vi "CallRosco_v2.vi"(6 "StopLV":bool, 8 "error in (no error)":errorcluster, 9 "ROSCO Params in":T3, 11 "ArrayPairs":T1={"iStatus"={"Index"=0, "Value"=0.0}, "TIME"={"Index"=1, "Value"=0.0}, "DT"={"Index"=2, "Value"=0.0}, "BL_PITCH"={"Index"=3, "Value"=0.0}, "VS_MECHGENPWR"={"Index"=13, "Value"=0.0}, "VS_GENPWR"={"Index"=14, "Value"=0.0}, "GEN_SPEED"={"Index"=19, "Value"=0.0}, "ROTOR_SPEED"={"Index"=20, "Value"=0.0}, "GENTQMEAS"={"Index"=22, "Value"=0.0}, "Y_M"={"Index"=23, "Value"=0.0}, "HORWINDV"={"Index"=26, "Value"=0.0}, "ROOTMOOP1"={"Index"=29, "Value"=0.0}, "ROOTMOOP2"={"Index"=30, "Value"=0.0}, "BL_PITCH2"={"Index"=32, "Value"=0.0}, "BL_PITCH3"={"Index"=33, "Value"=0.0}, "ROOTMOOP3"={"Index"=31, "Value"=0.0}, "AVCMSG_SIZE"={"Index"=48, "Value"=0.0}, "INFILE_SIZE "={"Index"=49, "Value"=0.0}, "OUTFILE_SIZE "={"Index"=50, "Value"=0.0}, "FA_ACC"={"Index"=52, "Value"=0.0}, "NUM_BLADES"={"Index"=60, "Value"=0.0}, "OUT_BL_PITCH"={"Index"=44, "Value"=0.0}, "OUT_TORQUE"={"Index"=46, "Value"=0.0}, "OUT_AERODYN_TQ"={"Index"=89, "Value"=0.0}}) -> (0 "error out":errorcluster, 1 "ROSCO Params out":T3, 4 "ArrayPairs 2":T1={"iStatus"={"Index"=0, "Value"=0.0}, "TIME"={"Index"=1, "Value"=0.0}, "DT"={"Index"=2, "Value"=0.0}, "BL_PITCH"={"Index"=3, "Value"=0.0}, "VS_MECHGENPWR"={"Index"=13, "Value"=0.0}, "VS_GENPWR"={"Index"=14, "Value"=0.0}, "GEN_SPEED"={"Index"=19, "Value"=0.0}, "ROTOR_SPEED"={"Index"=20, "Value"=0.0}, "GENTQMEAS"={"Index"=22, "Value"=0.0}, "Y_M"={"Index"=23, "Value"=0.0}, "HORWINDV"={"Index"=26, "Value"=0.0}, "ROOTMOOP1"={"Index"=29, "Value"=0.0}, "ROOTMOOP2"={"Index"=30, "Value"=0.0}, "BL_PITCH2"={"Index"=32, "Value"=0.0}, "BL_PITCH3"={"Index"=33, "Value"=0.0}, "ROOTMOOP3"={"Index"=31, "Value"=0.0}, "AVCMSG_SIZE"={"Index"=48, "Value"=0.0}, "INFILE_SIZE "={"Index"=49, "Value"=0.0}, "OUTFILE_SIZE "={"Index"=50, "Value"=0.0}, "FA_ACC"={"Index"=52, "Value"=0.0}, "NUM_BLADES"={"Index"=60, "Value"=0.0}, "OUT_BL_PITCH"={"Index"=44, "Value"=0.0}, "OUT_TORQUE"={"Index"=46, "Value"=0.0}, "OUT_AERODYN_TQ"={"Index"=89, "Value"=0.0}})   [LabVIEW 2018]
uses:
  Clusters/RoscoParams.ctl
  Clusters/ArrayPairs.ctl
  Clusters/SwapArrayCluster.ctl
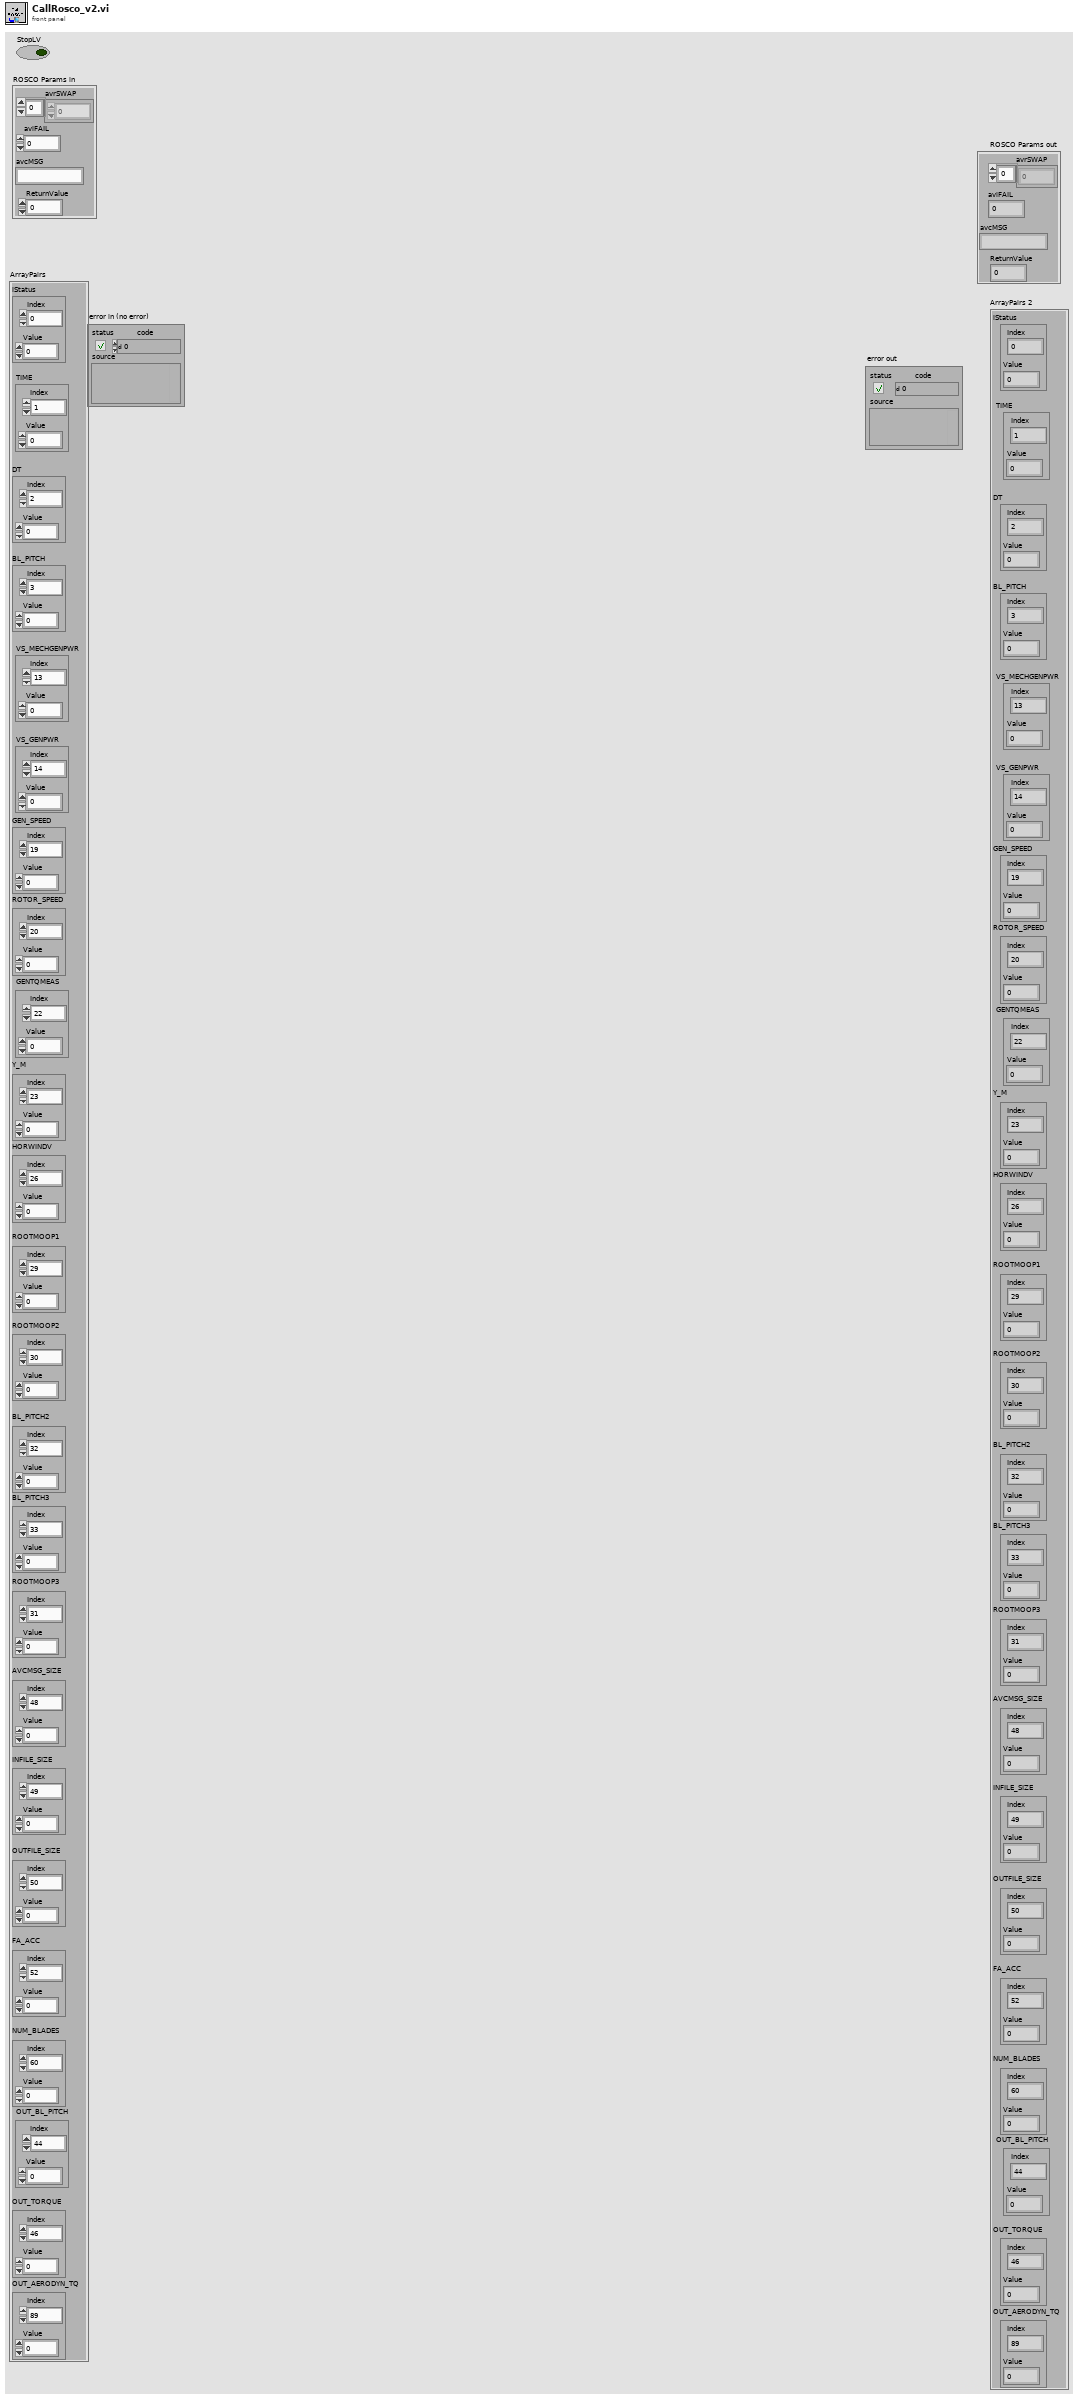
[diagram p1: front panel]
types:
  T1 = typedef "ArrayPairs.ctl" = cluster{"iStatus":T2, "TIME":T2, "DT":T2, "BL_PITCH":T2, "VS_MECHGENPWR":T2, "VS_GENPWR":T2, "GEN_SPEED":T2, "ROTOR_SPEED":T2, "GENTQMEAS":T2, "Y_M":T2, "HORWINDV":T2, "ROOTMOOP1":T2, "ROOTMOOP2":T2, "BL_PITCH2":T2, "BL_PITCH3":T2, "ROOTMOOP3":T2, "AVCMSG_SIZE":T2, "INFILE_SIZE ":T2, "OUTFILE_SIZE ":T2, "FA_ACC":T2, "NUM_BLADES":T2, "OUT_BL_PITCH":T2, "OUT_TORQUE":T2, "OUT_AERODYN_TQ":T2}
  T2 = typedef "SwapArrayCluster.ctl" = cluster{"Index":i32, "Value":sgl}
  T3 = typedef "RoscoParams.ctl" = cluster{"avrSWAP":sgl[], "aviFAIL":i32, "avcMSG":string, "ReturnValue":i32}
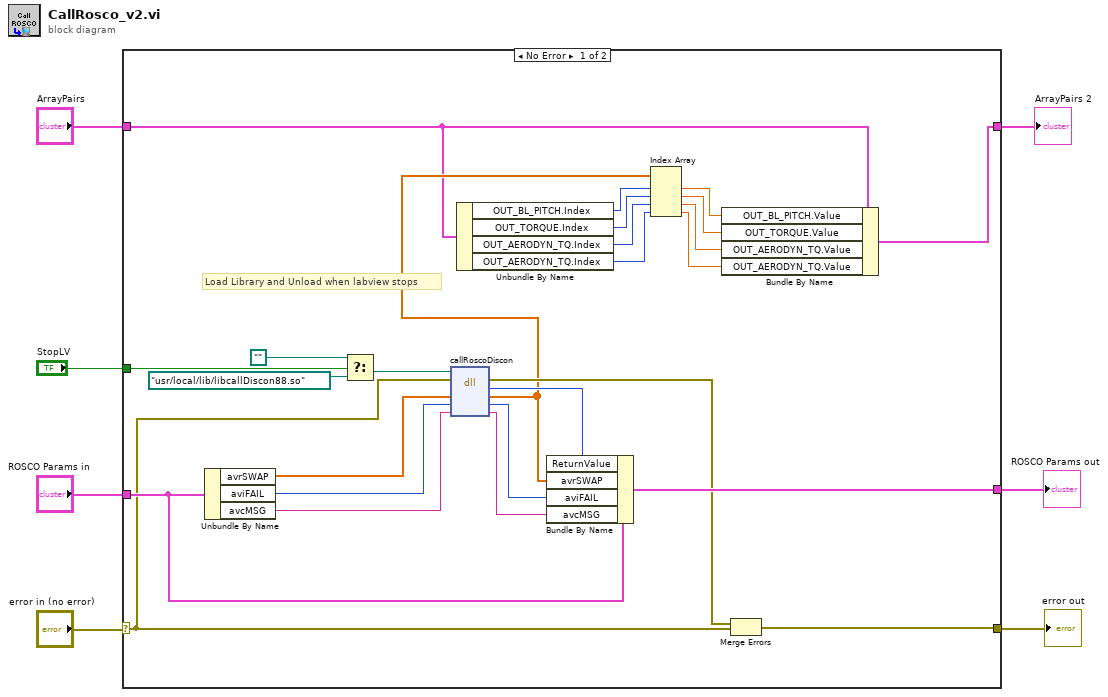
[diagram p0: block diagram]
diagram:
  n1 = case shown="No Error" "error in (no error)" {
    selector: "error in (no error)" -> [w19 w35]
    tunnel: [w32 w36] -> w7
    tunnel: "ROSCO Params in" -> [w31 w36]
    tunnel: "StopLV" -> [w29 _]
    tunnel: [w21 w35] -> w3
    tunnel: "ArrayPairs" -> [w14 w34]
    tunnel: [w10 w34] -> w1
    frame No Error {
      # "Load Library and Unload when labview stops"
      n2 = Unbundle By Name(w31) -> ("avrSWAP"=w28:sgl[], "aviFAIL"=w26:i32, "avcMSG"=w27:string)
      n3 = Select(t=path "", s=w29, f=path "/usr/local/lib/libcallDiscon88.so") -> (s? t:f=w25:path)
      n4 = dll-call lib="usr/local/lib/callDisconTest2.so" fn="callRoscoDiscon"(path in=w25, error in=w19, "avrSWAP"=w28, "aviFAIL"=w26, "arg3avcMSG"=w27) -> (error out=w20:errorcluster, "return type"=w22:i32, "avrSWAP"=w18:sgl[], "aviFAIL"=w33:i32, "arg3avcMSG"=w30:string)  [unwired: 1 in, 1 out]
      n5 = Unbundle By Name(w14) -> ("OUT_BL_PITCH.Index"=w17:i32, "OUT_TORQUE.Index"=w16:i32, "OUT_AERODYN_TQ.Index"=w15:i32, "OUT_AERODYN_TQ.Index"=w9:i32)
      n6 = Bundle By Name(cluster=w31, "ReturnValue"=w22, "avrSWAP"=w18, "aviFAIL"=w33, "avcMSG"=w30) -> (w32:T3)
      n7 = Index Array(array=w18, index #1=w17, index #2=w16, index #3=w15, index #4=w9) -> (element #1=w13:sgl, element #2=w12:sgl, element #3=w11:sgl, element #4=w8:sgl)
      n8 = Bundle By Name(cluster=w14, "OUT_BL_PITCH.Value"=w13, "OUT_TORQUE.Value"=w12, "OUT_AERODYN_TQ.Value"=w11, "OUT_AERODYN_TQ.Value"=w8) -> (w10:T1)
      n9 = Merge Errors(w20, w19) -> (w21:errorcluster)
    }
    frame Error {
    }
  }
  "ROSCO Params out" <- w7
  "error out" <- w3
  "ArrayPairs 2" <- w1
